vi "Combine Force Offsets.vi"(8 "error in (no error)":errorcluster) -> (0 "error out":errorcluster)   [LabVIEW 2013]
uses:
  Global Data/Transactions/Dataset Source.ctl
  Global Data/Transactions/Dataset Transaction Id.ctl
  Global Data/Transactions/Dataset Type.ctl
  Apps/Yes No Button.ctl
  Data Access Objects/Metadata/DAO Actions.ctl
  Data Access Objects/Metadata/DAO Actions with Remove.ctl
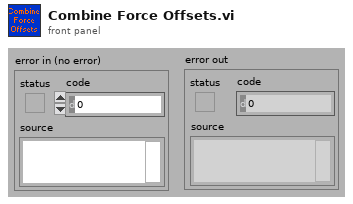
[diagram p1: front panel]
types:
  T1 = typedef "DAO Actions.ctl" = enum16{"Init", "Get", "Set"}
  T2 = typedef "Dataset Type.ctl" = enum16{"LVDT", "Load Cell", "Actuator Command", "Servo Error", "Displacement Command", "Displacement", "Force"}
  T3 = typedef "Dataset Transaction Id.ctl" = cluster{"Dataset Source":T4, "Dataset Type":T2, "Hold":T5, "Volts":T5, "Tag":string}
  T4 = typedef "Dataset Source.ctl" = enum16{"LBCB 1", "LBCB 2", "Combined", "External Sensors"}
  T5 = typedef "Yes No Button.ctl" = bool
  T6 = typedef "DAO Actions with Remove.ctl" = enum16{"Init", "Get", "Set", "Remove"}
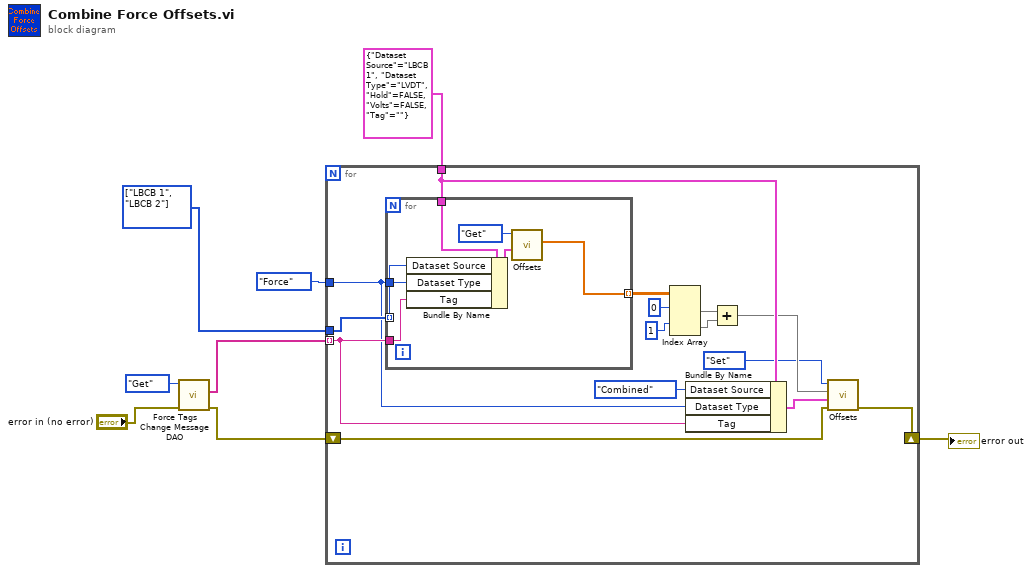
[diagram p0: block diagram]
diagram:
  w7 = T4[] [enum."LBCB 1", enum."LBCB 2"] items=["LBCB 1", "LBCB 2", "Combined", "External Sensors"]
  n1 = call "Force Tags Change Message DAO.vi"("error in (no error)"="error in (no error)", "DAO Actions"=DAO_Actions."Get") -> ("error out"=w2:errorcluster, "Force Tags"=w4:string[])  [unwired: 7 in, 1 out]
  n2 = for {
    tunnel: T3 {"Dataset Source"=enum."LBCB 1", "Dataset Type"=enum."LVDT", "Hold"=FALSE, "Volts"=FALSE, "Tag"=""} ("Dataset Trans Id") -> [w22]
    tunnel: w7 -> [w23]
    tunnel: Dataset_Type."Force" ("Dataset Type") -> [w9]
    tunnel: w4 -> [w15] mode=indexing
    shift-right: [w13] -> w1
    shift-left: w2 -> [w14]
    n3 = for {
      tunnel: w22 -> [w30]
      tunnel: w23 -> [w28] mode=indexing
      tunnel: [w27] -> w21 mode=indexing
      tunnel: w9 -> [w26]
      tunnel: w15 -> [w24]
      n4 = Bundle By Name(cluster=w30, "Dataset Source"=w28, "Dataset Type"=w26, "Tag"=w24) -> (w29:T3)
      n5 = call "Offsets.vi"("Dataset Trans Id"=w29, "DAO Actions"=DAO_Actions_with_Remove."Get") -> ("Data Out"=w27:dbl[])  [unwired: 7 in, 2 out]
    }
    n6 = Index Array(array=w21, index (row) #1=0 ("index (row)"), index (row) #2=1 ("index (row)")) -> (element #1=w18:dbl[], element #2=w17:dbl[])  [unwired: 2 in]
    n7 = Bundle By Name(cluster=w22, "Dataset Source"=Dataset_Source."Combined", "Dataset Type"=w9, "Tag"=w15) -> (w12:T3)
    n8 = Add(x=w18, y=w17) -> (x+y=w16:dbl[])
    n9 = call "Offsets.vi"("error in (no error)"=w14, "Dataset Trans Id"=w12, "Data In"=w16, "DAO Actions"=DAO_Actions_with_Remove."Set") -> ("error out"=w13:errorcluster)  [unwired: 5 in, 2 out]
  }
  "error out" <- w1
